vi "Pre Launch Init.vi"(11 "Mediator in":refnum<class "Mediator.lvclass">) -> (0 "error out":errorcluster, 3 "Mediator out":refnum<class "Mediator.lvclass">)   [LabVIEW 2015, in "Mediator.lvlib" / "Mediator.lvclass"]
doc: "(<B>Filename</B>: Actor Framework.lvlib:Actor.lvclass:Pre Launch Init.vi)\n\nDefines behavior that occurs after the Launch Nested Actor method is invoked but before the actor's Actor Core method begins running.\n\nBy default, this method does nothing. A descendant class may override it to define behavior."
uses:
  Mediator.lvclass
  TopicLookupTable/TopicLookupTable.lvclass
  Mediator.lvclass/Mediator.ctl
  IMediator/IMediator/IMediator.lvclass/IMediator.ctl
  <vilib>/ActorFramework/Actor/Actor.lvclass/Actor.ctl
  <vilib>/ActorFramework/Message Enqueuer/Message Enqueuer.lvclass/Message Enqueuer.ctl
  IMediator/IMediator Messages/Start Bus Monitor Msg/Start Bus Monitor Msg.lvclass/Start Bus Monitor Msg.ctl
  <vilib>/ActorFramework/Message Enqueuer/Enqueue.vi
  <vilib>/ActorFramework/Message Enqueuer/Init from Existing Queue.vi
  <vilib>/ActorFramework/Message Priority Queue/Priority Enqueue.vi
  IMediator/IMediator/IMediator.lvclass
  IMediator/IMediator Messages/Start Bus Monitor Msg/Start Bus Monitor Msg.lvclass
  <vilib>/ActorFramework/Message Enqueuer/Message Enqueuer.lvclass
  <vilib>/ActorFramework/Actor/Actor.lvclass
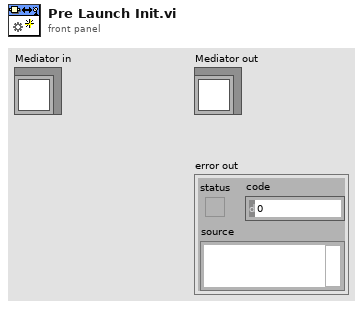
[diagram p1: front panel]
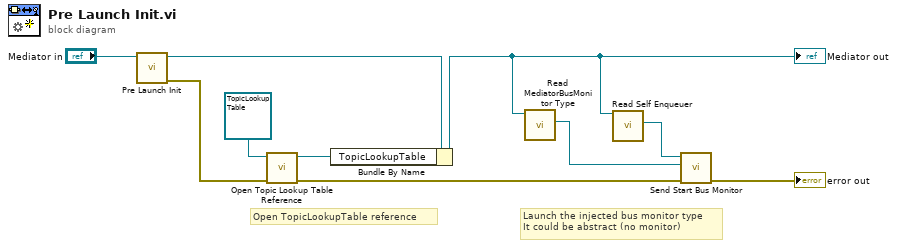
[diagram p0: block diagram]
diagram:
  # "Launch the injected bus monitor type\nIt could be abstract (no monitor)"
  # "Open TopicLookupTable reference"
  n1 = call-parent "Pre Launch Init.vi"("Actor in"="Mediator in") -> ("error out"=w7:errorcluster, "Actor out"=w10:refnum<class "Mediator.lvclass">)  [unwired: 9 in]
  n2 = call "Open Topic Lookup Table Reference.vi"("error in (no error)"=w7, "TopicLookupTable in"=refnum<class "TopicLookupTable.lvclass"> refnum ("Mediator.lvlib:TopicLookupTable.lvclass")) -> ("error out"=w6:errorcluster, "TopicLookupTable Reference"=w8:refnum<data-value>)  [unwired: 8 in]
  n3 = Bundle By Name(cluster=w10, "TopicLookupTable"=w8) -> (w2:refnum<class "Mediator.lvclass">)
  "Mediator out" <- w2
  n4 = call "Read MediatorBusMonitor Type.vi"("IMediator in"=w2) -> ("MediatorBusMonitor (Type)"=w3:refnum<class "IMediatorBusMonitor.lvclass">)  [unwired: 10 in]
  n5 = call <vilib>:"Read Self Enqueuer.vi"("Actor"=w2) -> ("Self Enqueuer"=w1:refnum<class "Message Enqueuer.lvclass">)  [unwired: 10 in]
  n6 = call "Send Start Bus Monitor.vi"("error in (no error)"=w6, "MediatorBusMonitor (Type)"=w3, "Message Enqueuer"=w1) -> ("error out"=→"error out":errorcluster)  [unwired: 7 in, 1 out]
